vi "Write Velocity.vi"(10 "Velocity":T1, 11 "Movable in":refnum<class "Movable.lvclass">) -> (3 "Movable out":refnum<class "Movable.lvclass">)   [LabVIEW 2021, in "Movable.lvclass"]
doc: "MIT Licence\nCopyright (c) 2024 David Grollier"
uses:
  Movable.lvclass
  Type Def/Velocity.ctl
  Movable.lvclass/Movable.ctl
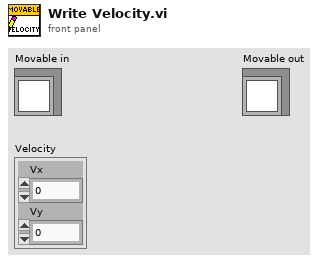
[diagram p1: front panel]
types:
  T1 = typedef "Velocity.ctl" = cluster{"Vx":dbl, "Vy":dbl}
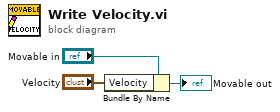
[diagram p0: block diagram]
diagram:
  n1 = Bundle By Name(cluster="Movable in", "Velocity"="Velocity") -> (→"Movable out":refnum<class "Movable.lvclass">)
